vi "showRfItems.vi"(8 "error in (no error)":errorcluster, 10 "show/hide":bool, 11 "StaticOutputEditor in":refnum<class "StaticOutputEditor.lvclass">) -> (0 "error out":errorcluster, 3 "StaticOutputEditor out":refnum<class "StaticOutputEditor.lvclass">)   [LabVIEW 2011, in "Views.lvlib" / "ScriptEditor.lvlib" / "StaticOutputEditor.lvclass"]
uses:
  StaticOutputEditor.lvclass
  StaticOutputEditor.lvclass/StaticOutputEditor.ctl
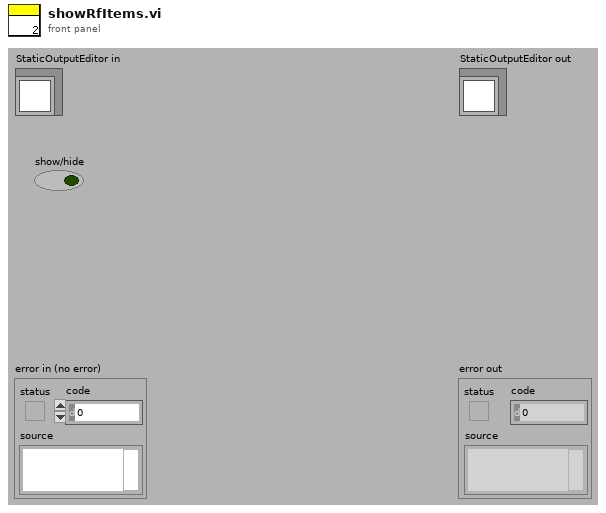
[diagram p1: front panel]
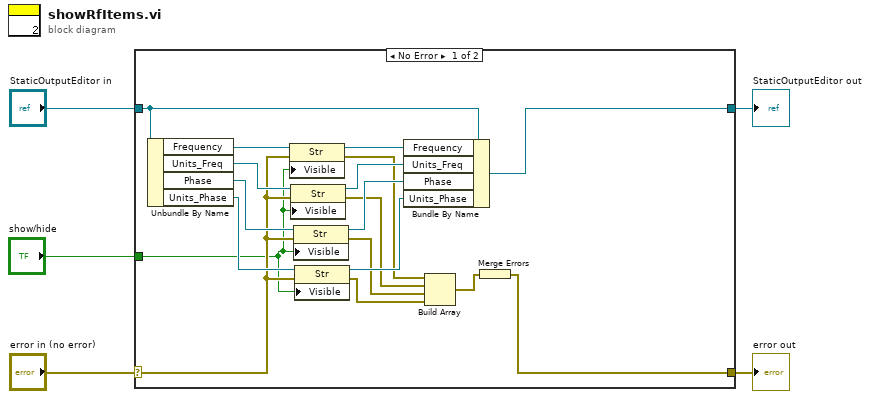
[diagram p0: block diagram]
diagram:
  n1 = case shown="No Error" "error in (no error)" {
    selector: "error in (no error)" -> [w19 w25]
    tunnel: [w6 w25] -> w4
    tunnel: [w16 w24] -> w2
    tunnel: "StaticOutputEditor in" -> [w17 w24]
    tunnel: "show/hide" -> [w18 _]
    frame No Error {
      n2 = Unbundle By Name(w17) -> ("Frequency"=w23:refnum<vi>, "Units_Freq"=w22:refnum<vi>, "Phase"=w21:refnum<vi>, "Units_Phase"=w20:refnum<vi>)
      n3 = property class="Str"(reference=w23, error in=w19, "Visible"=w18) -> (reference out=w15:refnum<vi>, error out=w11:errorcluster)
      n4 = property class="Str"(reference=w22, error in=w19, "Visible"=w18) -> (reference out=w14:refnum<vi>, error out=w10:errorcluster)
      n5 = property class="Str"(reference=w21, error in=w19, "Visible"=w18) -> (reference out=w13:refnum<vi>, error out=w9:errorcluster)
      n6 = property class="Str"(reference=w20, error in=w19, "Visible"=w18) -> (reference out=w12:refnum<vi>, error out=w8:errorcluster)
      n7 = Bundle By Name(cluster=w17, "Frequency"=w15, "Units_Freq"=w14, "Phase"=w13, "Units_Phase"=w12) -> (w16:refnum<class "StaticOutputEditor.lvclass">)
      n8 = Build Array(w11, w10, w9, w8) -> (w7:errorcluster[])
      n9 = Merge Errors(w7) -> (w6:errorcluster)
    }
    frame Error {
    }
  }
  "error out" <- w4
  "StaticOutputEditor out" <- w2
